vi "New BS120x Device.vi"   [LabVIEW 2021, in "BS120x Driver.lvlib"]
uses:
  BS120x Driver.lvlib
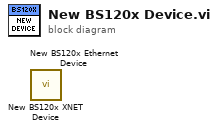
[diagram p0: block diagram]
diagram:
  n1 = call "New BS120x XNET Device.vi"() -> ()  [unwired: 10 in, 2 out]
  n2 = call "New BS120x Ethernet Device.vi"() -> ()  [unwired: 10 in, 2 out]
